vi "adcmt6243_inst.vi"() -> ()   [LabVIEW 2020]
panel:
  out "Voltage":dbl
  out "Measure Unit":string
  out "Voltage Chart":dbl(graph)
  out "Current":dbl(graph)
  out "Current":dbl
  out "Time remaining (s)":dbl
  out "Finished":bool
  out "Elapsed Time (s)":dbl
  out "Unit":string
  in  "Reset":bool
  in  "Stop":bool
  in  "Start":bool
  in  "Set value":bool
  in  "time":dbl
  in  "voltage":dbl
  in  "current":dbl
  in  "GPIB address":u16
  in  "Check":bool
  in  "stop (forced)":bool
  out "Query Data":string
  # "Check connection"
  # "Output monitor"
  # "Setting"
  # "Current"
  # "mA"
  # "Voltage"
  # "V"
  # "Time"
  # "seconds"
  # "Operation"
  # "Monitor"
  # "seconds"
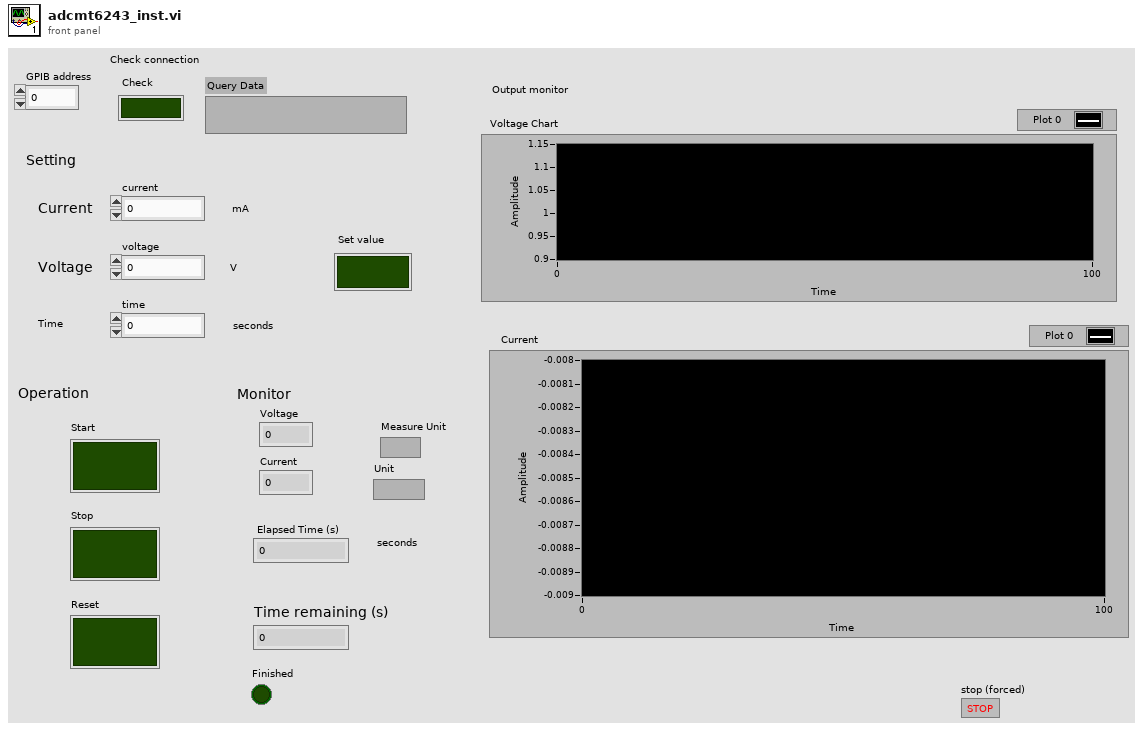
[diagram p1: front panel]
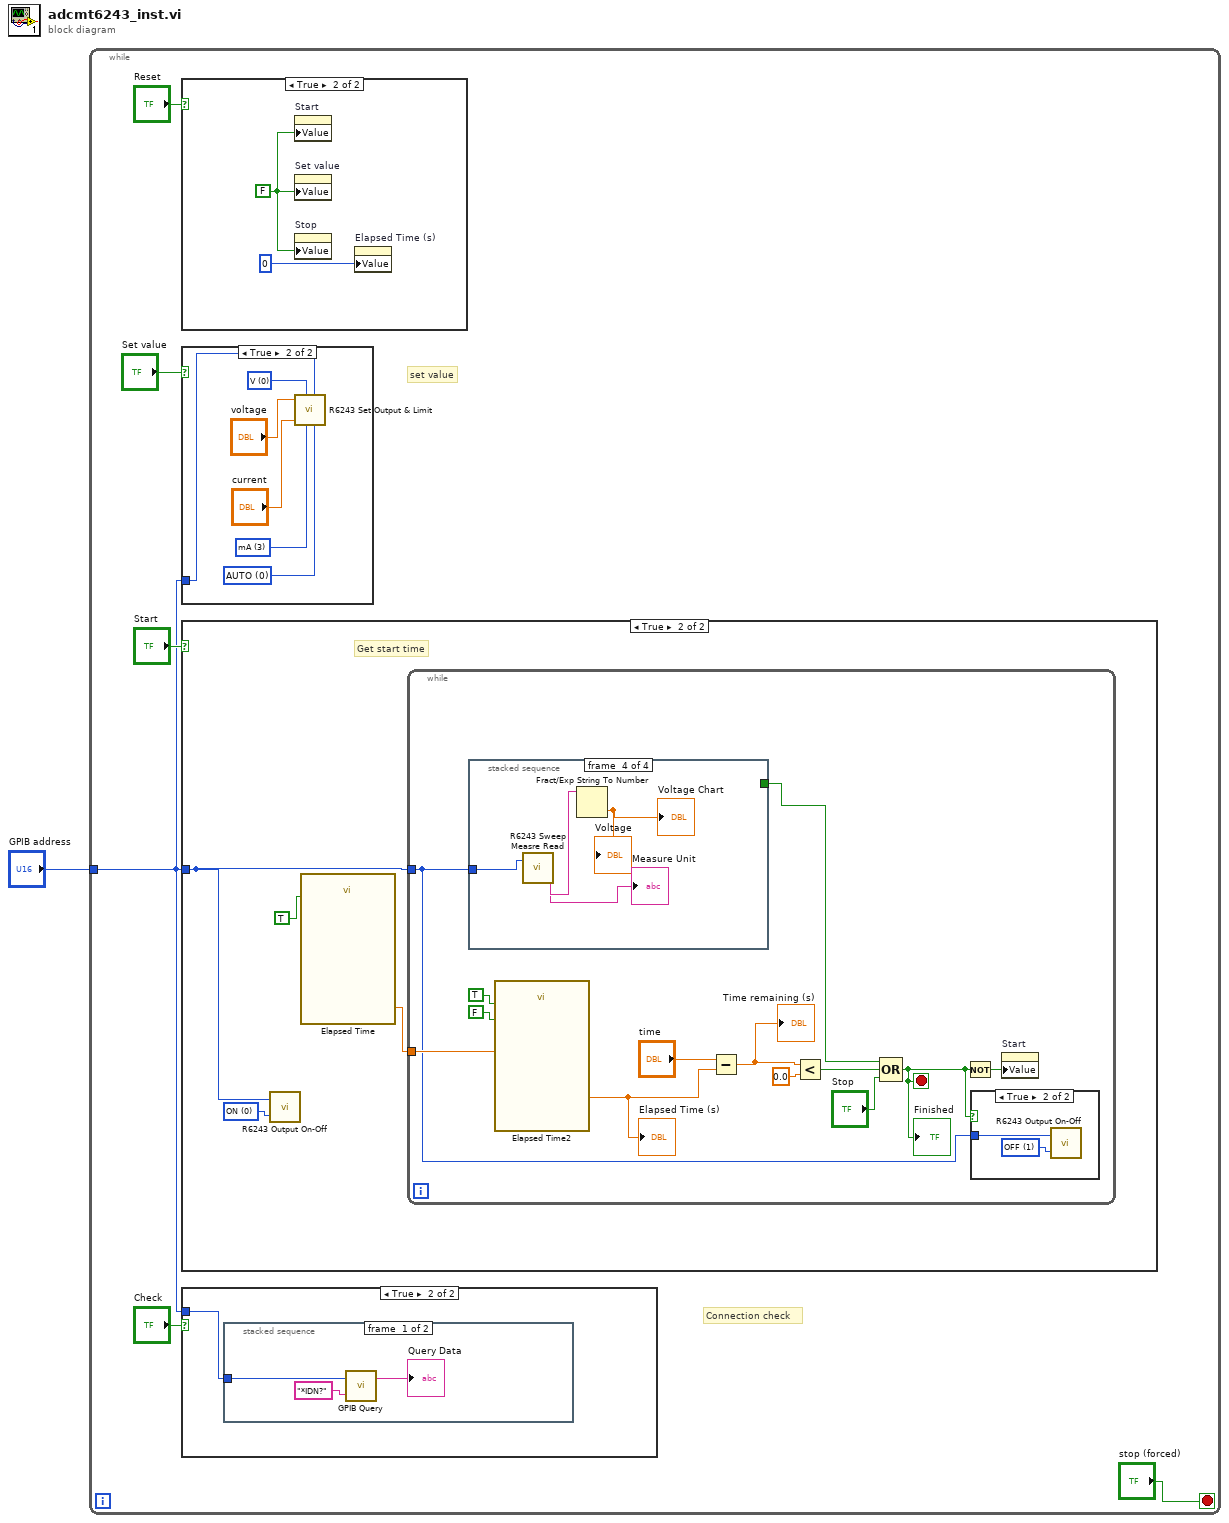
[diagram p0: block diagram]
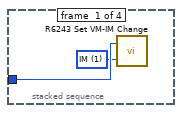
[diagram p3: hidden frame]
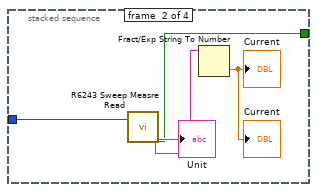
[diagram p4: hidden frame]
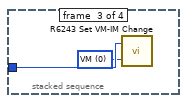
[diagram p5: hidden frame]
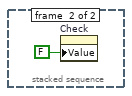
[diagram p10: hidden frame]
diagram:
  n1 = while {
    tunnel: "GPIB address" -> [w2]
    stop <- "stop (forced)" stop-if-true
    # "Connection check"
    # "set value"
    n2 = case shown="True" "Reset" {
      frame False {
      }
      frame True {
        w41 = FALSE ("Start")
        n3 = property on="Start" class="Bool (strict)"("Value"=w41) -> ()  [unwired: 2 in, 2 out]
        n4 = property on="Set value" class="Bool (strict)"("Value"=w41) -> ()  [unwired: 2 in, 2 out]
        n5 = property on="Stop" class="Bool (strict)"("Value"=w41) -> ()  [unwired: 2 in, 2 out]
        n6 = property on="Elapsed Time (s)" class="DigNum (strict)"("Value"=0) -> ()  [unwired: 2 in, 2 out]
      }
    }
    n7 = case shown="True" "Set value" {
      tunnel: w2 -> [_ w44]
      frame False {
      }
      frame True {
        w42 = u16 0 items=["V", "mV", "A", "mA", "uA"] ("Unit_O")
        w43 = u16 3 items=["V", "mV", "A", "mA", "uA"] ("Unit_L")
        w47 = u16 0 items=["AUTO", "FIX"] ("Range Mode")
        n8 = call <instrlib>:"R6243 Set Output & Limit.vi"("Output"="voltage", "Unit_O"=w42, "Limit"="current", "Unit_L"=w43, "GPIB Address"=w44, "Range Mode"=w47) -> ()  [unwired: 4 in, 1 out]
      }
    }
    n9 = case shown="True" "Start" {
      tunnel: w2 -> [_ w10]
      frame False {
      }
      frame True {
        w11 = u16 0 items=["ON", "OFF"] ("Output")
        # "Get start time"
        n10 = call <instrlib>:"R6243 Output On-Off.vi"("Output"=w11, "GPIB Address"=w10) -> ()  [unwired: 1 out]
        n11 = call "Elapsed Time"("Reset"=TRUE) -> ("Present (s)"=w9:dbl)  [unwired: 11 in, 7 out]
        n12 = while {
          tunnel: w10 -> [w14]
          tunnel: w9 -> [w24]
          stop <- w13 stop-if-true
          n13 = stacked-sequence {
            tunnel: w14 -> [w26 w31 w33 w35]
            tunnel: [_ w29 _ _] -> w12
            frame #0 {
              w25 = u16 1 items=["VM", "IM"] ("Measure Func.")
              n14 = call <instrlib>:"R6243 Set VM-IM Change.vi"("Measure Func."=w25, "Address"=w26) -> ()  [unwired: 1 out]
            }
            frame #1 {
              n15 = call <instrlib>:"R6243 Sweep Measre Read.vi"("GPIB Address"=w31) -> ("GPIB Error"=w29:bool, "Data Str"=w28:string, "Measure Unit"=→"Unit":string)  [unwired: 4 out]
              n16 = Fract/Exp String To Number(string=w28) -> (number=→"Current" →"Current":dbl)  [unwired: 3 in, 1 out]
            }
            frame #2 {
              w32 = u16 0 items=["VM", "IM"] ("Measure Func.")
              n17 = call <instrlib>:"R6243 Set VM-IM Change.vi"("Measure Func."=w32, "Address"=w33) -> ()  [unwired: 1 out]
            }
            frame #3 {
              n18 = call <instrlib>:"R6243 Sweep Measre Read.vi"("GPIB Address"=w35) -> ("Data Str"=w37:string, "Measure Unit"=→"Measure Unit":string)  [unwired: 5 out]
              n19 = Fract/Exp String To Number(string=w37) -> (number=→"Voltage Chart" →"Voltage":dbl)  [unwired: 3 in, 1 out]
            }
          }
          n20 = call "Elapsed Time2"("Reset"=TRUE, "Auto Reset"=FALSE, "Set Start Time (s)"=w24) -> ("Elapsed Time (s)"=w22:dbl)  [unwired: 9 in, 7 out]
          "Elapsed Time (s)" <- w22
          n21 = Subtract(x="time", y=w22) -> (x-y=w15:dbl)
          "Time remaining (s)" <- w15
          n22 = Less?(x=w15, y=0.0) -> (x < y?=w17:bool)
          n23 = Compound Arithmetic op=OR(w12, w17, "Stop") -> (w13:bool)
          "Finished" <- w13
          n24 = Not(x=w13) -> (.not. x?=w20:bool)
          n25 = case shown="True" w13 {
            tunnel: w14 -> [_ w38]
            frame False {
            }
            frame True {
              w39 = u16 1 items=["ON", "OFF"] ("Output")
              n26 = call <instrlib>:"R6243 Output On-Off.vi"("Output"=w39, "GPIB Address"=w38) -> ()  [unwired: 1 out]
            }
          }
          n27 = property on="Start" class="Bool (strict)"("Value"=w20) -> ()  [unwired: 2 in, 2 out]
        }
      }
    }
    n28 = case shown="True" "Check" {
      tunnel: w2 -> [_ w48]
      frame False {
      }
      frame True {
        n29 = stacked-sequence {
          tunnel: w48 -> [w49 _]
          frame #0 {
            n30 = call <instrlib>:"GPIB Query.vi"("Command String"="*IDN?", "Address"=w49) -> ("Query Data"=→"Query Data":string)  [unwired: 1 out]
          }
          frame #1 {
            n31 = property on="Check" class="Bool (strict)"("Value"=FALSE ("Boolean")) -> ()  [unwired: 2 in, 2 out]
          }
        }
      }
    }
  }
